vi "TDT-Open Tank.vi"(0 "Data":T1={"TTankX"=refnum, "TDevAccX"=refnum, "LastTime"=0.0, "error"={"status"=FALSE, "code"=0, "source"=""}, "Block Name"="", "Circuit Tag"="", "Tank Name"="", "NumTicks"=0, "LastTick"=0.0, "Idle?"=FALSE, "Wait (ms)"=1000, "LastArtf"=0.0, "LastTosc"=0.0}, 11 "error in (no error)":errorcluster) -> (4 "Data (out)":T1={"TTankX"=refnum, "TDevAccX"=refnum, "LastTime"=0.0, "error"={"status"=FALSE, "code"=0, "source"=""}, "Block Name"="", "Circuit Tag"="", "Tank Name"="", "NumTicks"=0, "LastTick"=0.0, "Idle?"=FALSE, "Wait (ms)"=1000, "LastArtf"=0.0, "LastTosc"=0.0}, 15 "error out":errorcluster)   [LabVIEW 2015]
uses:
  TDT Interface Data.ctl
  TDT-Sys Mode Enum.ctl
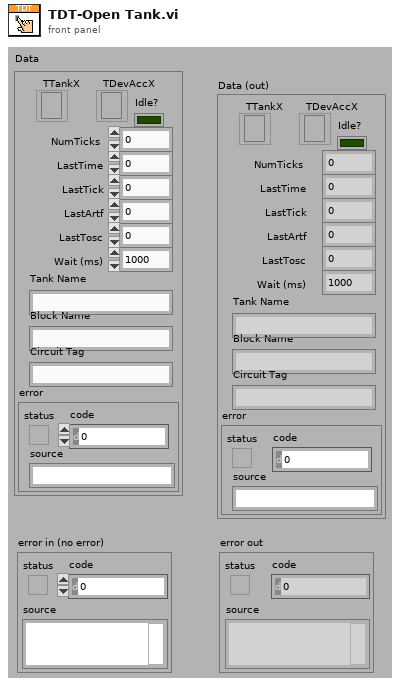
[diagram p1: front panel]
types:
  T1 = typedef "TDT Interface Data.ctl" = cluster{"TTankX":refnum<k7>, "TDevAccX":refnum<k7>, "LastTime":dbl, "error":errorcluster, "Block Name":string, "Circuit Tag":string, "Tank Name":string, "NumTicks":i32, "LastTick":dbl, "Idle?":bool, "Wait (ms)":u32, "LastArtf":dbl, "LastTosc":dbl}
  T2 = typedef "TDT-Sys Mode Enum.ctl" = enum16{"Idle", "Standby", "Preview", "Record"}
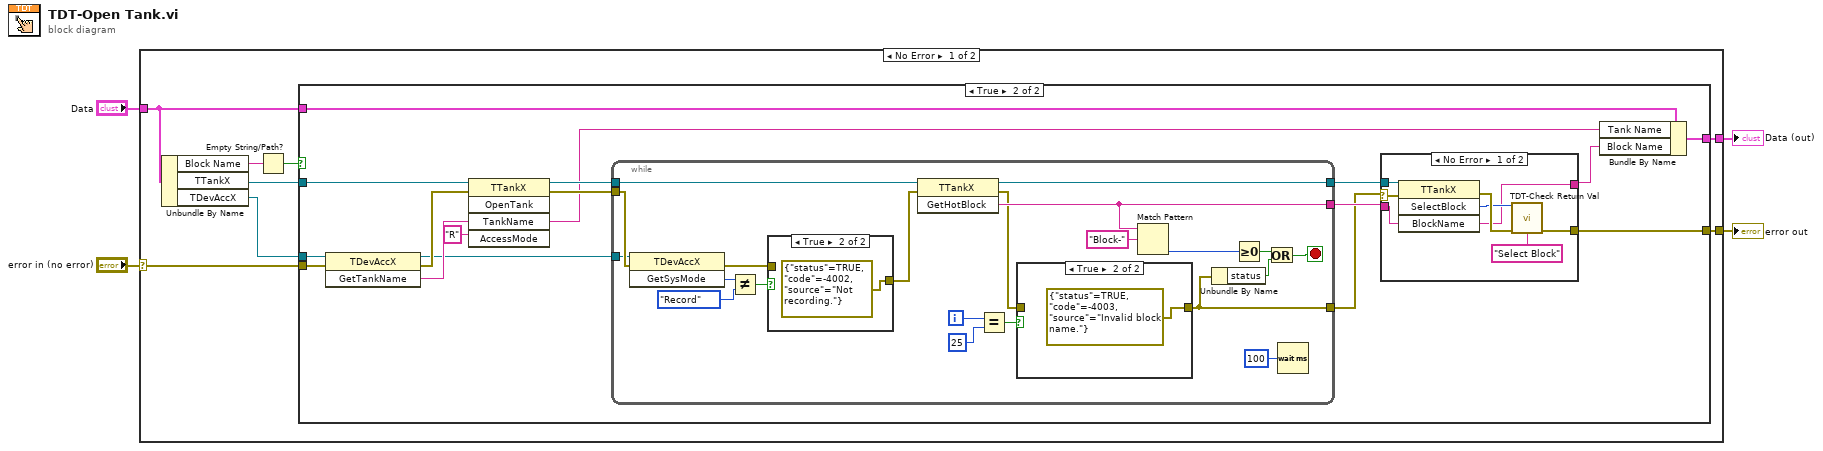
[diagram p0: block diagram]
diagram:
  n1 = case shown="No Error" "error in (no error)" {
    selector: "error in (no error)" -> [w11 w67]
    tunnel: [w12 w67] -> w3
    tunnel: "Data" -> [w8 w66]
    tunnel: [w7 w66] -> w1
    frame No Error {
      n2 = Unbundle By Name(w8) -> ("Block Name"=w5:string, "TTankX"=w9:refnum<k7>, "TDevAccX"=w10:refnum<k7>)
      n3 = Empty String/Path?(string/path=w5) -> (empty?=w6:bool)
      n4 = case shown="True" w6 {
        tunnel: [w14 w31] -> w12
        tunnel: w11 -> [w14 w30]
        tunnel: w10 -> [_ w27]
        tunnel: w9 -> [_ w26]
        tunnel: w8 -> [w13 w18]
        tunnel: [w13 w15] -> w7
        frame False {
        }
        frame True {
          n5 = invoke class="TDevAccX" method="GetTankName"(reference=w27, error in=w30) -> (reference out=w19:refnum<k7>, error out=w23:errorcluster, "GetTankName"=w24:string)  [unwired: 1 in]
          n6 = invoke class="TTankX" method="OpenTank"(reference=w26, error in=w23, "TankName"=w24, "AccessMode"="R") -> (reference out=w25:refnum<k7>, error out=w21:errorcluster, "TankName"=w17:string)  [unwired: 1 in, 2 out]
          n7 = while {
            tunnel: [w61] -> w29
            tunnel: [w58] -> w28
            tunnel: w25 -> [w60]
            tunnel: w21 -> [w47]
            tunnel: [w48] -> w20
            tunnel: w19 -> [w46]
            i -> [w55]
            stop <- w52 stop-if-true
            n8 = invoke class="TDevAccX" method="GetSysMode"(reference=w46, error in=w47) -> (error out=w42:errorcluster, "GetSysMode"=w45:i32)  [unwired: 1 in, 1 out]
            n9 = Not Equal?(x=w45, y=TDT-Sys_Mode_Enum."Record" ("Mode")) -> (x != y?=w43:bool)
            n10 = case shown="True" w43 {
              tunnel: w42 -> [w62 _]
              tunnel: [w62 errorcluster {"status"=TRUE, "code"=-4002, "source"="Not recording."} ("error out")] -> w41
              frame False {
              }
              frame True {
              }
            }
            n11 = invoke class="TTankX" method="GetHotBlock"(reference=w60, error in=w41) -> (reference out=w61:refnum<k7>, error out=w50:errorcluster, "GetHotBlock"=w58:string)  [unwired: 1 in]
            n12 = Equal?(x=w55, y=25) -> (x = y?=w51:bool)
            n13 = case shown="True" w51 {
              tunnel: w50 -> [w64 _]
              tunnel: [w64 errorcluster {"status"=TRUE, "code"=-4003, "source"="Invalid block name."} ("error out")] -> w48
              frame False {
              }
              frame True {
              }
            }
            n14 = Match Pattern(string=w58, regular expression="Block-") -> (offset past match=w56:i32)  [unwired: 1 in, 3 out]
            n15 = Unbundle By Name(w48) -> ("status"=w49:bool)
            n16 = Greater Or Equal To 0?(x=w56) -> (x >= 0?=w53:bool)
            n17 = Or(x=w53, y=w49) -> (x .or. y?=w52:bool)
            n18 = Wait (ms)(milliseconds to wait=u32 100) -> ()  [unwired: 1 out]
          }
          n19 = case shown="No Error" w20 {
            selector: w20 -> [w32 w40]
            tunnel: [w38 w40] -> w31
            tunnel: w29 -> [w37 _]
            tunnel: w28 -> [w36 _]
            tunnel: [w33 _] -> w16
            frame No Error {
              n20 = invoke class="TTankX" method="SelectBlock"(reference=w37, error in=w32, "BlockName"=w36) -> (error out=w35:errorcluster, "SelectBlock"=w34:i32, "BlockName"=w33:string)  [unwired: 1 in, 1 out]
              n21 = call "TDT-Check Return Val.vi"("Return Val"=w34, "error in (no error)"=w35, "source"="Select Block" ("Message")) -> ("error out"=w38:errorcluster)  [unwired: 12 in]
            }
            frame Error {
            }
          }
          n22 = Bundle By Name(cluster=w18, "Tank Name"=w17, "Block Name"=w16) -> (w15:T1)
        }
      }
    }
    frame Error {
    }
  }
  "error out" <- w3
  "Data (out)" <- w1
